vi "Terminal_PressureSyetem_Work_Condition.vi"(11 "液压子系统监测参数":T1) -> (3 "达到工作条件":bool)   [LabVIEW 2014]
uses:
  Work_Condition.vi
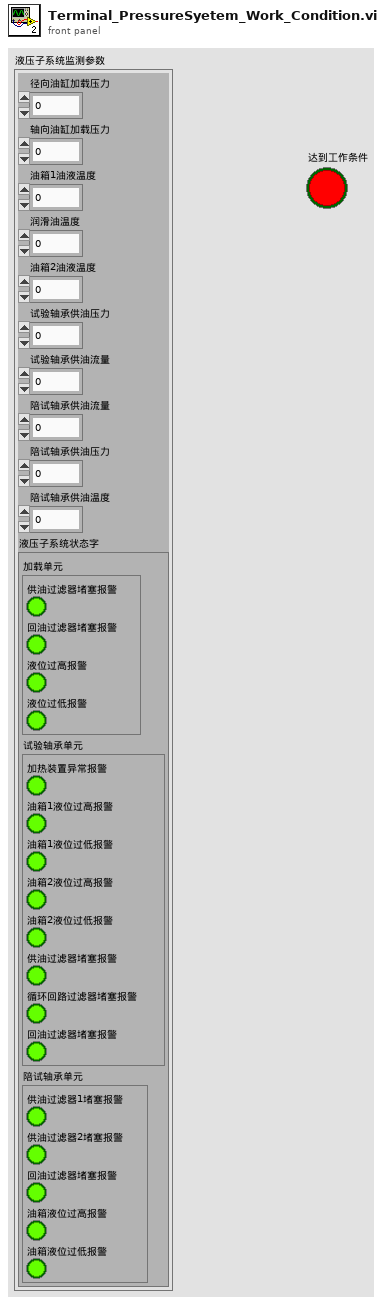
[diagram p1: front panel]
types:
  T1 = cluster{"径向油缸加载压力":u16, "轴向油缸加载压力":u16, "油箱1油液温度":u16, "润滑油温度":u16, "油箱2油液温度":u16, "试验轴承供油压力":u16, "试验轴承供油流量":u16, "陪试轴承供油流量":u16, "陪试轴承供油压力":u16, "陪试轴承供油温度":u16, "液压子系统状态字":cluster{"加载单元":cluster{"供油过滤器堵塞报警":bool, "回油过滤器堵塞报警":bool, "液位过高报警":bool, "液位过低报警":bool}, "试验轴承单元":cluster{"加热装置异常报警":bool, "油箱1液位过高报警":bool, "油箱1液位过低报警":bool, "油箱2液位过高报警":bool, "油箱2液位过低报警":bool, "供油过滤器堵塞报警":bool, "循环回路过滤器堵塞报警":bool, "回油过滤器堵塞报警":bool}, "陪试轴承单元":cluster{"供油过滤器1堵塞报警":bool, "供油过滤器2堵塞报警":bool, "回油过滤器堵塞报警":bool, "油箱液位过高报警":bool, "油箱液位过低报警":bool}}}
  T2 = cluster{"加载单元":cluster{"供油过滤器堵塞报警":bool, "回油过滤器堵塞报警":bool, "液位过高报警":bool, "液位过低报警":bool}, "试验轴承单元":cluster{"加热装置异常报警":bool, "油箱1液位过高报警":bool, "油箱1液位过低报警":bool, "油箱2液位过高报警":bool, "油箱2液位过低报警":bool, "供油过滤器堵塞报警":bool, "循环回路过滤器堵塞报警":bool, "回油过滤器堵塞报警":bool}, "陪试轴承单元":cluster{"供油过滤器1堵塞报警":bool, "供油过滤器2堵塞报警":bool, "回油过滤器堵塞报警":bool, "油箱液位过高报警":bool, "油箱液位过低报警":bool}}
  T3 = cluster{"供油过滤器堵塞报警":bool, "回油过滤器堵塞报警":bool, "液位过高报警":bool, "液位过低报警":bool}
  T4 = cluster{"加热装置异常报警":bool, "油箱1液位过高报警":bool, "油箱1液位过低报警":bool, "油箱2液位过高报警":bool, "油箱2液位过低报警":bool, "供油过滤器堵塞报警":bool, "循环回路过滤器堵塞报警":bool, "回油过滤器堵塞报警":bool}
  T5 = cluster{"供油过滤器1堵塞报警":bool, "供油过滤器2堵塞报警":bool, "回油过滤器堵塞报警":bool, "油箱液位过高报警":bool, "油箱液位过低报警":bool}
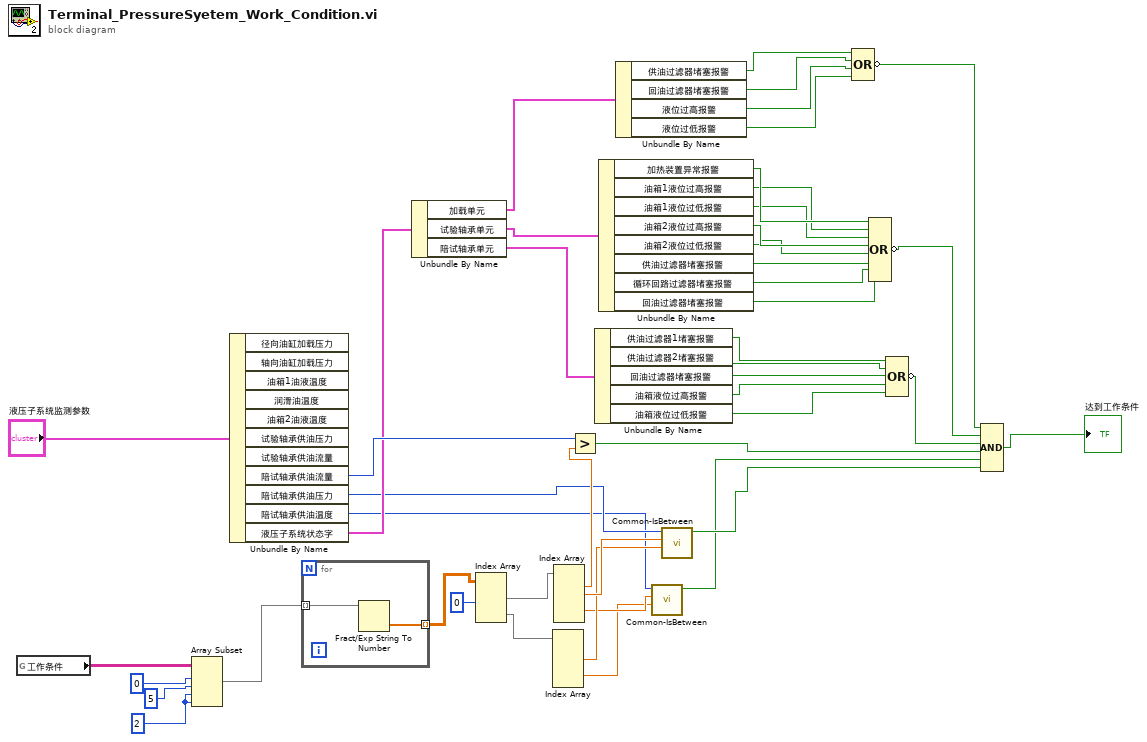
[diagram p0: block diagram]
diagram:
  w46 = 2
  n1 = global read "Work_Condition.vi" "工作条件"() -> (w11:string[][])
  n2 = Array Subset(array=w11, index (row)=0, length (row)=5, index (col)=w46, length (col)=w46) -> (w43:string[][])
  n3 = Unbundle By Name("液压子系统监测参数") -> ("陪试轴承供油流量"=w44:u16, "陪试轴承供油压力"=w10:u16, "陪试轴承供油温度"=w6:u16, "液压子系统状态字"=w36:T2)  [unwired: 7 out]
  n4 = for {
    tunnel: w43 -> [w48] mode=indexing
    tunnel: [w47] -> w42 mode=indexing
    n5 = Fract/Exp String To Number(string=w48) -> (number=w47:dbl[])  [unwired: 3 in, 1 out]
  }
  n6 = Unbundle By Name(w36) -> ("加载单元"=w35:T3, "试验轴承单元"=w34:T4, "陪试轴承单元"=w33:T5)
  n7 = Index Array(array=w42, index (col) #1=0) -> (element #1=w40:dbl[], element #2=w38:dbl[])  [unwired: 3 in]
  n8 = Index Array(array=w38) -> (element #2=w8:dbl, element #4=w4:dbl)  [unwired: 5 in, 3 out]
  n9 = Index Array(array=w40) -> (element #1=w39:dbl, element #2=w9:dbl, element #4=w5:dbl)  [unwired: 5 in, 2 out]
  n10 = Greater?(x=w44, y=w39) -> (0:w37:bool)
  n11 = Unbundle By Name(w33) -> ("供油过滤器1堵塞报警"=w20:bool, "供油过滤器2堵塞报警"=w19:bool, "回油过滤器堵塞报警"=w18:bool, "油箱液位过高报警"=w17:bool, "油箱液位过低报警"=w16:bool)
  n12 = Unbundle By Name(w34) -> ("加热装置异常报警"=w28:bool, "油箱1液位过高报警"=w27:bool, "油箱1液位过低报警"=w26:bool, "油箱2液位过高报警"=w25:bool, "油箱2液位过低报警"=w24:bool, "供油过滤器堵塞报警"=w23:bool, "循环回路过滤器堵塞报警"=w22:bool, "回油过滤器堵塞报警"=w21:bool)
  n13 = Unbundle By Name(w35) -> ("供油过滤器堵塞报警"=w32:bool, "回油过滤器堵塞报警"=w31:bool, "液位过高报警"=w30:bool, "液位过低报警"=w29:bool)
  n14 = call "Common-IsBetween.vi"("比例(0.1)"=w4, "基数"=w5, "x"=w6) -> ("范围内？"=w1:bool)  [unwired: 8 in]
  n15 = call "Common-IsBetween.vi"("比例(0.1)"=w8, "基数"=w9, "x"=w10) -> ("范围内？"=w7:bool)  [unwired: 8 in]
  n16 = Compound Arithmetic op=OR(w32, w31, w30, w29) -> (invert w15:bool)
  n17 = Compound Arithmetic op=OR(w28, w27, w26, w25, w24, w23, w22, w21) -> (invert w14:bool)
  n18 = Compound Arithmetic op=OR(w20, w19, w18, w17, w16) -> (invert w13:bool)
  n19 = Compound Arithmetic op=AND(w15, w14, w13, w37, w1, w7) -> (→"达到工作条件":bool)
